vi "Get User Interfaces.vi"(11 "Component in":refnum<class "Component.lvclass">) -> (2 "User Interfaces":refnum<class "Component User Interfaces.lvclass">, 3 "Component out":refnum<class "Component.lvclass">)   [LabVIEW 2017, in "DSF Core.lvlib" / "Component.lvclass"]
uses:
  Component.lvclass
  Component User Interface/Component User Interfaces.lvclass
  Component.lvclass/Component.ctl
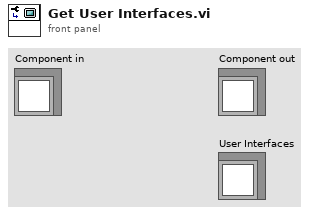
[diagram p1: front panel]
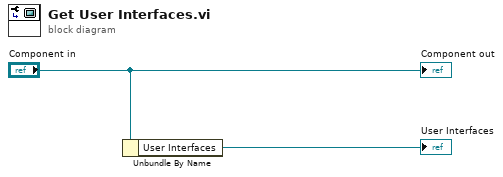
[diagram p0: block diagram]
diagram:
  n1 = Unbundle By Name("Component in") -> ("User Interfaces"=→"User Interfaces":refnum<class "Component User Interfaces.lvclass">)
  "Component out" <- "Component in"
